vi "GetHeaderValue.vi"(1 "Server Frame":T1, 3 "Header Name":string, 5 "error in":errorcluster) -> (15 "Value":string, 19 "error out":errorcluster)   [LabVIEW 2017, in "LabVIEW STOMP.lvlib" / "STOMP.lvclass"]
uses:
  STOMP.lvclass
  Typedefs/Type_ServerFrame.ctl
  Typedefs/Type_ServerFrameType.ctl
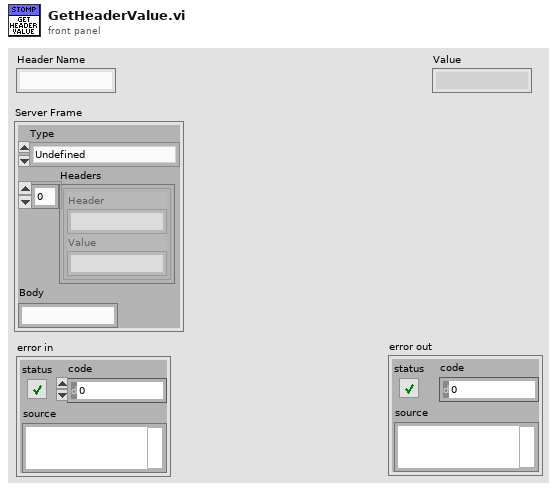
[diagram p1: front panel]
types:
  T1 = typedef "LabVIEW STOMP.lvlib/STOMP.lvclass/Type_ServerFrame.ctl" = cluster{"Type":T2, "Headers":cluster{"Header":string, "Value":string}[], "Body":string}
  T2 = typedef "LabVIEW STOMP.lvlib/STOMP.lvclass/Type_ServerFrameType.ctl" = enum16{"Undefined", "MESSAGE", "CONNECTED", "RECEIPT", "ERROR"}
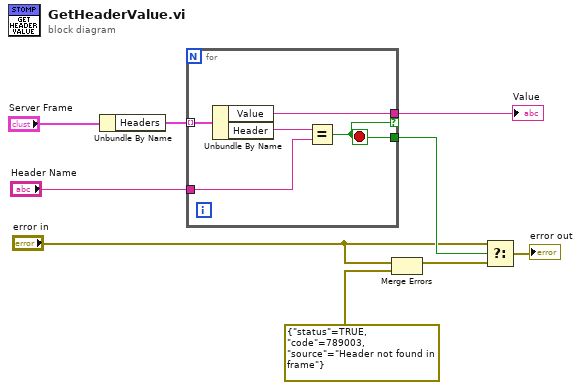
[diagram p0: block diagram]
diagram:
  n1 = Unbundle By Name("Server Frame") -> ("Headers"=w8:cluster{"Header":string, "Value":string}[])
  n2 = for {
    tunnel: w8 -> [w14] mode=indexing
    tunnel: "Header Name" -> [w12]
    tunnel: [w11] -> w6 if=w10
    tunnel: [w10] -> w5
    stop <- w10 stop-if-true
    n3 = Unbundle By Name(w14) -> ("Value"=w11:string, "Header"=w13:string)
    n4 = Equal?(x=w13, y=w12) -> (x = y?=w10:bool)
  }
  "Value" <- w6
  n5 = Merge Errors("error in", errorcluster {"status"=TRUE, "code"=789003, "source"="Header not found in frame"} ("error constant")) -> (w2:errorcluster)
  n6 = Select(t="error in", s=w5, f=w2) -> (s? t:f=→"error out":errorcluster)
